vi "Setup Test Log.vi"(8 "error in (no error)":errorcluster, 10 "Model in":refnum<class "Model.lvclass">, 11 "Boot Loader in":refnum<class "Boot Loader.lvclass">) -> (0 "error out":errorcluster, 2 "Model out":refnum<class "Model.lvclass">, 3 "Boot Loader out":refnum<class "Boot Loader.lvclass">)   [LabVIEW 2016, in "Boot Loader.lvclass"]
uses:
  Boot Loader.lvclass
  Model/Model.lvclass
  Typedefs/TestLogTypes.ctl
  Test Log/Test Log Factory/Test Log Factory.lvclass
  Model/Model.lvclass/Model.ctl
  Typedefs/HPMT_Typedefs.lvlib
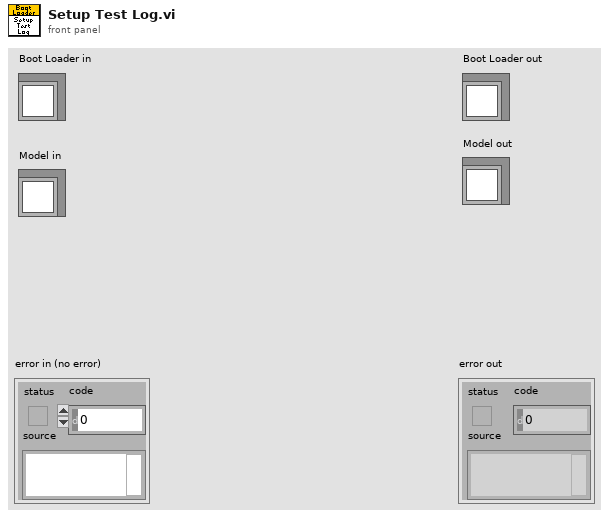
[diagram p1: front panel]
types:
  T1 = typedef "HPMT_Typedefs.lvlib/TestLogTypes.ctl" = enum16{"CSV Test Log"}
  T2 = typedef "HPMT_Typedefs.lvlib/TestSettings.ctl" = cluster{"Operator":string, "Strut Number":string, "Test Stand Serial Number":string, "Notes":string, "Test Angle":u16, "Number of Cycles":u16, "Data Points per Cycle":u16, "Settling Time (secs)":u16, "Breakaway Air Pressure":u16, "Largest Strut Displacement":dbl, "Load Cell Sensitivity":dbl}
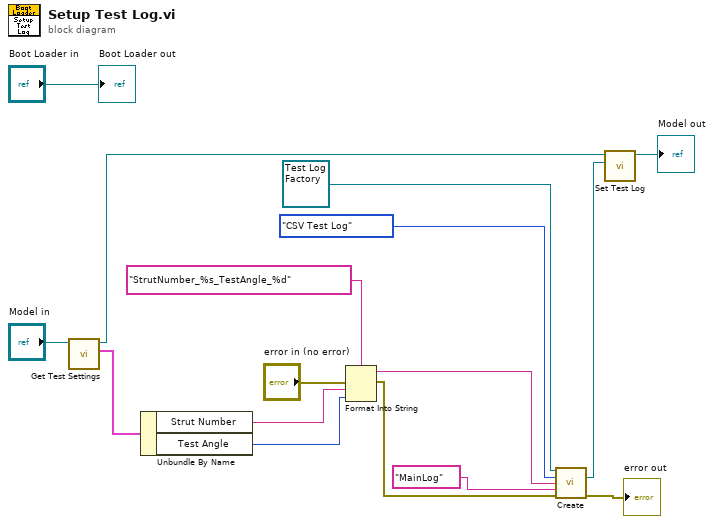
[diagram p0: block diagram]
diagram:
  n1 = call "Get Test Settings.vi"("Model in"="Model in") -> ("Test Settings"=w12:T2, "Model out"=w10:refnum<class "Model.lvclass">)  [unwired: 9 in]
  n2 = Unbundle By Name(w12) -> ("Strut Number"=w4:string, "Test Angle"=w3:u16)
  n3 = Format Into String(format string="StrutNumber_%s_TestAngle_%d", error in="error in (no error)", w4, w3) -> (resulting string=w7:string, error out=w2:errorcluster)  [unwired: 1 in]
  n4 = call-dynamic "Create.vi"("Test Log Factory in"=refnum<class "Test Log Factory.lvclass"> refnum ("Test Log Factory.lvclass"), "Test Log Types"=TestLogTypes."CSV Test Log" ("TestLogTypes"), "Test Name"=w7, "Scan Name"="MainLog", "error in (no error)"=w2) -> ("Test Log"=w15:refnum<class "Test Log.lvclass">, "error out"=→"error out":errorcluster)  [unwired: 8 in, 1 out]
  n5 = call "Set Test Log.vi"("ITestLog.lvclass"=w15, "Model in"=w10) -> ("Model out"=→"Model out":refnum<class "Model.lvclass">)  [unwired: 9 in]
  "Boot Loader out" <- "Boot Loader in"
